vi "SwerveJoystickLogic.vi"(7 "Gyro":dbl, 8 "TankMode":bool, 10 "Joystick Axes":dbl[](array[numeric])) -> (2 "Speeds":dbl[](array[numeric]), 3 "Angles":dbl[](array[numeric]))   [LabVIEW 2019]
uses:
  Robot Global Data.vi
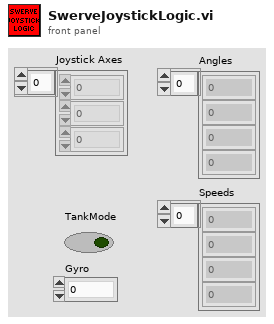
[diagram p1: front panel]
types:
  T1 = typedef "WPI_DriverStationRobotMode2.ctl" = enum16{"Autonomous Disabled", "Autonomous Enabled", "Teleop Disabled", "Teleop Enabled", "Disconnected", "Finish", "Test Disabled", "Test Enabled", "Emergency Stopped"}
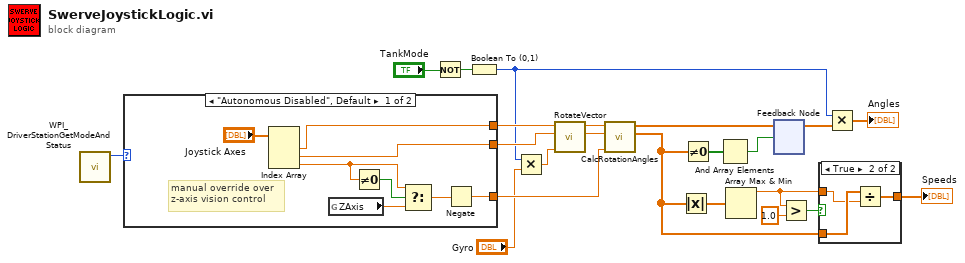
[diagram p0: block diagram]
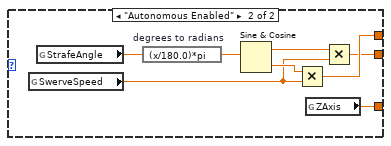
[diagram p2: hidden frame]
diagram:
  n1 = call <vilib>:"WPI_DriverStationGetModeAndStatus.vi"() -> ("Robot Mode"=w3:T1)  [unwired: 10 in, 1 out]
  n2 = case shown="\"Autonomous Disabled\", Default" w3 {
    tunnel: [w23 w33] -> w14
    tunnel: [w25 w32] -> w13
    tunnel: [w24 w31] -> w2
    frame "Autonomous Disabled", Default {
      # "manual override over\nz-axis vision control"
      n3 = Index Array(array="Joystick Axes") -> (element #1=w23:dbl, element #2=w25:dbl, element #3=w26:dbl)  [unwired: 3 in]
      n4 = global read "Robot Global Data.vi" "ZAxis"() -> (w27:dbl)
      n5 = Not Equal To 0?(x=w26) -> (x != 0?=w28:bool)
      n6 = Select(t=w26, s=w28, f=w27) -> (s? t:f=w29:dbl)
      n7 = Negate(x=w29) -> (-x=w24:dbl)
    }
    frame "Autonomous Enabled" {
      n8 = global read "Robot Global Data.vi" "SwerveSpeed"() -> (w34:dbl)
      n9 = global read "Robot Global Data.vi" "StrafeAngle"() -> (w38:dbl)
      n10 = expression code="(x/180.0)*pi" "degrees to radians"(w38) -> (w37:dbl)
      n11 = Sine & Cosine(0:w37) -> (1:w36:dbl, 2:w35:dbl)
      n12 = Multiply(x=w35, y=w34) -> (x*y=w33:dbl)
      n13 = global read "Robot Global Data.vi" "ZAxis"() -> (w31:dbl)
      n14 = Multiply(x=w36, y=w34) -> (x*y=w32:dbl)
    }
  }
  n15 = Not(x="TankMode") -> (.not. x?=w8:bool)
  n16 = Boolean To (0,1)(Boolean=w8) -> (0, 1=w4:i16)
  n17 = Multiply(x=w4, y="Gyro") -> (x*y=w7:dbl)
  n18 = call "RotateVector.vi"("Angle"=w7, "Y"=w13, "X"=w14) -> ("Y'"=w10:dbl, "X'"=w11:dbl)  [unwired: 6 in]
  n19 = call "CalcRotationAngles.vi"("ZAxis"=w2, "YAxis"=w10, "XAxis"=w11) -> ("Speeds"=w18:dbl[], "Angles"=w17:dbl[])  [unwired: 7 in]
  n20 = Absolute Value(x=w18) -> (abs(x)=w19:dbl[])
  n21 = Not Equal To 0?(x=w18) -> (x != 0?=w12:bool[])
  n22 = And Array Elements(Boolean array=w12) -> (logical AND=w16:bool)
  n23 = Array Max & Min(array=w19) -> (max value=w20:dbl)  [unwired: 3 out]
  n24 = feedback #1() -> (w6:dbl[])  [unwired: 1 in]
  n25 = feedback-in #1(w17, w16) -> ()
  n26 = Greater?(x=w20, y=1.0) -> (0:w22:bool)
  n27 = case shown="True" w22 {
    tunnel: w18 -> [w39 w42]
    tunnel: w20 -> [_ w41]
    tunnel: [w39 w40] -> w15
    frame False {
    }
    frame True {
      n28 = Divide(x=w42, y=w41) -> (x/y=w40:dbl[])
    }
  }
  "Speeds" <- w15
  n29 = Multiply(x=w4, y=w6) -> (x*y=→"Angles":dbl[])
